vi "LV2GlobalArray.vi"(3 "Index":i32, 4 "Write":dbl[](array[numeric]) format="%.2f", 5 "Mode":T1(ring)) -> (1 "Read":dbl[](array[numeric]) format="%.2f", 2 "Read one":dbl format="%.2f")   [LabVIEW 2016]
doc: "Demo of LV2 style global variable.\n\n\nMode :\n - Initialize : creates the array (size and values defined by Write)\n - Write : replaces a given number of elements of the array (number and values defined\n by Write, start index defined by Index)\n - Read : reads the whole array --> Read\n - Read one : read the element defined by Index --> Read one"
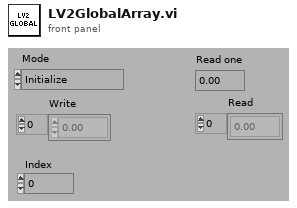
[diagram p1: front panel]
types:
  T1 = enum16{"Initialize", "Write", "Read all", "Read one"}
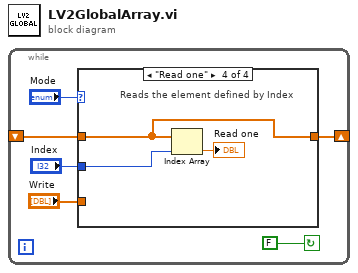
[diagram p0: block diagram]
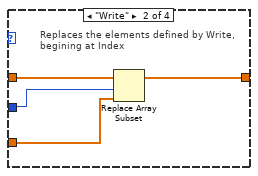
[diagram p3: hidden frame]
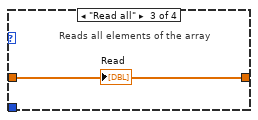
[diagram p4: hidden frame]
diagram:
  n1 = while {
    shift-right: [w5] -> _
    shift-left: _ -> [w3]
    stop <- FALSE continue-if-true
    n2 = case shown="\"Read one\"" "Mode" {
      tunnel: [w7 w10 w12 w13] -> w5
      tunnel: w3 -> [_ w11 w12 w13]
      tunnel: "Index" -> [_ w9 _ w15]
      tunnel: "Write" -> [w7 w8 _ _]
      frame "Initialize", Default {
        # "Initializes the shift register with\nthe values defined by Write"
      }
      frame "Write" {
        # "Replaces the elements defined by Write,\nbegining at Index"
        n3 = Replace Array Subset(array=w11, new element=w8, index=w9) -> (w10:dbl[])
      }
      frame "Read all" {
        # "Reads all elements of the array"
        "Read" <- w12
      }
      frame "Read one" {
        # "Reads the element defined by Index"
        n4 = Index Array(array=w13, index=w15) -> (element=→"Read one":dbl)
      }
    }
  }
